vi "TestVision_v1.vi"() -> ()   [LabVIEW 2019]
uses:
  <vilib>/userDefined/High Color/IMAQdx.ctl
  <vilib>/vision/driver/NI_Vision_Acquisition_Software.lvlib
panel:
  out "Image 2":T1(plugin-control)
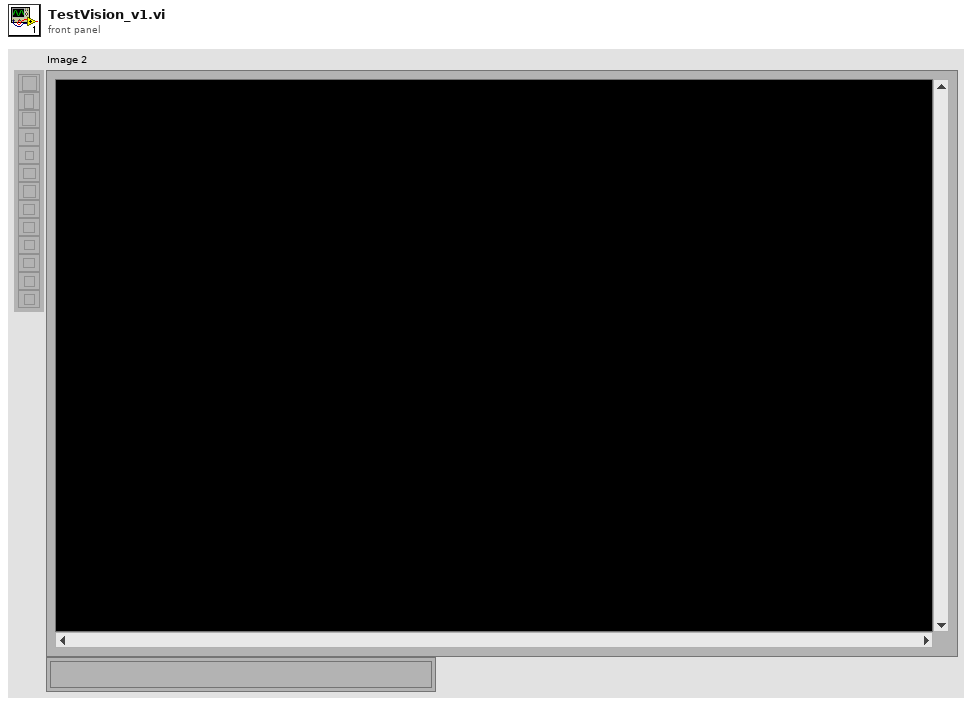
[diagram p1: front panel]
types:
  T1 = typedef "IMAQ Image.ctl" = refnum<image>
  T2 = typedef "IMAQdx.ctl" = refnum<k21>
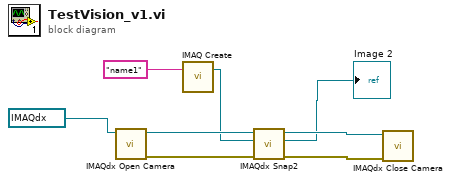
[diagram p0: block diagram]
diagram:
  n1 = call <vilib>:"IMAQdx Open Camera.vi"("Session In"=T2 "cam0") -> ("error out"=w6:errorcluster, "Session Out"=w8:T2)  [unwired: 9 in]
  n2 = call "IMAQ Create"("Image Name"="name1") -> ("New Image"=w3:T1)  [unwired: 4 in, 1 out]
  n3 = call <vilib>:"IMAQdx Snap2.vi"("error in"=w6, "Image In"=w3, "Session In"=w8) -> ("error out"=w5:errorcluster, "Image Out"=→"Image 2":T1, "Session Out"=w7:T2)  [unwired: 6 in]
  n4 = call <vilib>:"IMAQdx Close Camera.vi"("error in"=w5, "Session In"=w7) -> ()  [unwired: 9 in, 1 out]
